vi "util.load.test.cases.vi"(11 "String":string) -> (3 "Array":T1[](array[typedef]))   [LabVIEW 2021]
uses:
  Test.Case.type.ctl
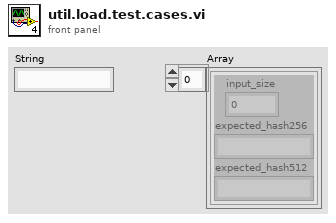
[diagram p1: front panel]
types:
  T1 = typedef "Test.Case.type.ctl" = cluster{"input_size":i32, "expected_hash256":string, "expected_hash512":string}
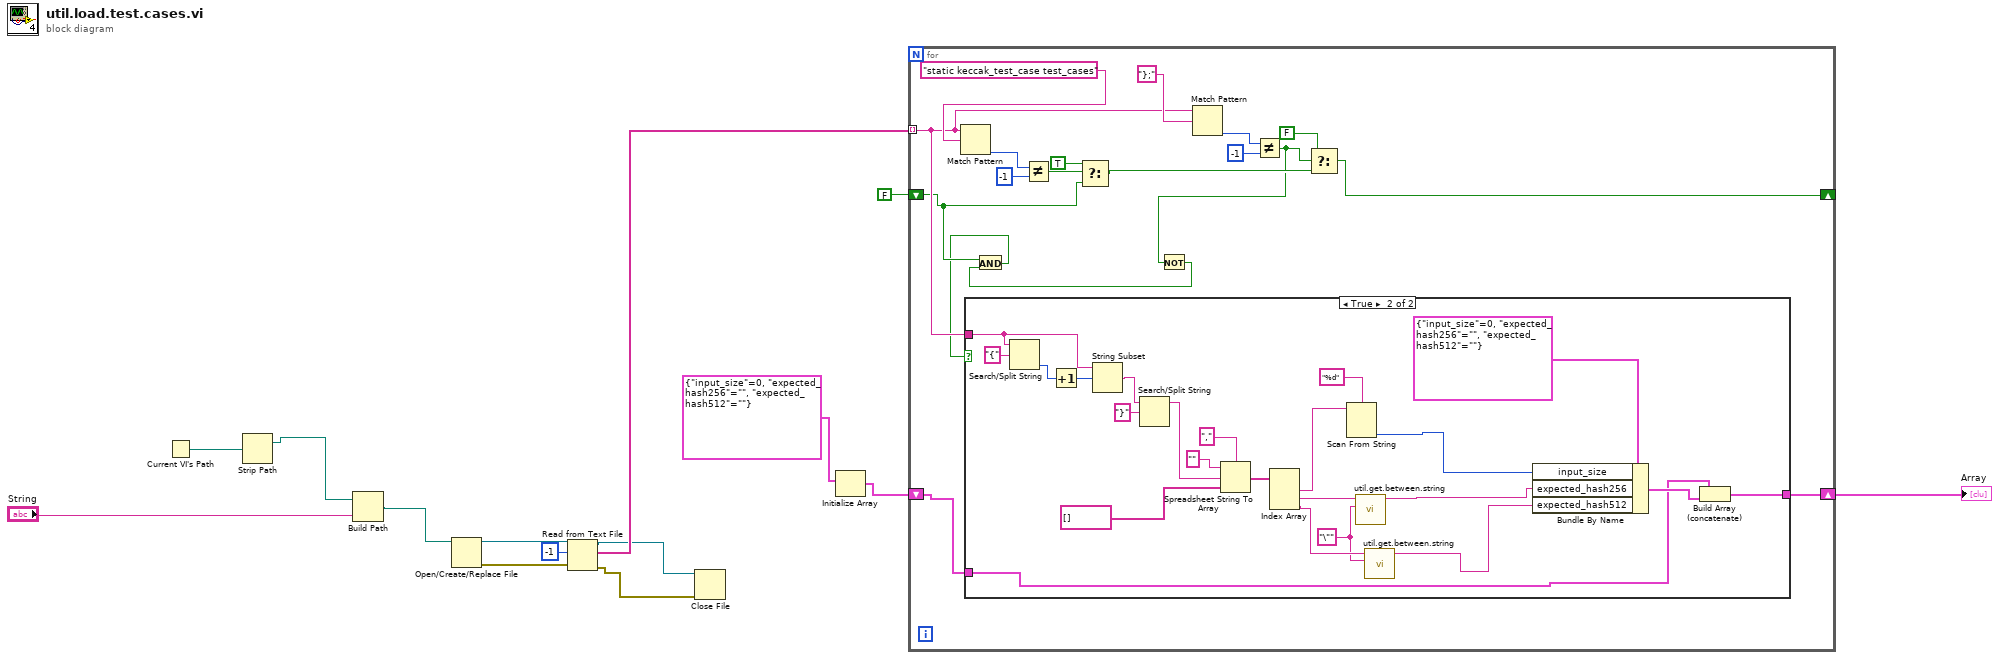
[diagram p0: block diagram]
diagram:
  n1 = Current VI's Path() -> (path=w7:path)
  n2 = Strip Path(path=w7) -> (stripped path=w8:path)  [unwired: 1 out]
  n3 = Build Path(base path=w8, name or relative path="String") -> (appended path=w2:path)
  n4 = Open/Create/Replace File(file path (use dialog)=w2) -> (refnum out=w3:refnum<file>, error out=w5:errorcluster)  [unwired: 5 in, 1 out]
  n5 = Read from Text File(file (use dialog)=w3, count=-1, error in=w5) -> (refnum out=w4:refnum<file>, text=w10:string[], error out=w6:errorcluster)  [unwired: 1 in, 1 out]
  n6 = Close File(refnum=w4, error in=w6) -> ()  [unwired: 2 out]
  n7 = Initialize Array(T1 {"input_size"=0, "expected_hash256"="", "expected_hash512"=""}) -> (w12:T1[])  [unwired: 1 in]
  n8 = for {
    tunnel: w10 -> [w26] mode=indexing
    shift-right: [w22] -> _
    shift-left: FALSE -> [w20]
    shift-right: [w16] -> w14
    shift-left: w12 -> [w15]
    n9 = Match Pattern(string=w26, regular expression="static keccak_test_case test_cases") -> (offset past match=w31:i32)  [unwired: 1 in, 3 out]
    n10 = Not Equal?(x=w31, y=-1) -> (x != y?=w29:bool)
    n11 = Select(t=TRUE, s=w29, f=w20) -> (s? t:f=w23:bool)
    n12 = Match Pattern(string=w26, regular expression="};") -> (offset past match=w25:i32)  [unwired: 1 in, 3 out]
    n13 = Not Equal?(x=w25, y=-1) -> (x != y?=w18:bool)
    n14 = Not(x=w18) -> (.not. x?=w17:bool)
    n15 = And(x=w20, y=w17) -> (x .and. y?=w19:bool)
    n16 = case shown="True" w19 {
      tunnel: w26 -> [_ w53]
      tunnel: [w33 w35] -> w16
      tunnel: w15 -> [w33 w34]
      frame False {
      }
      frame True {
        w41 = "\"" ("search string/char (-)")
        n17 = Search/Split String(string=w53, search string/char (-)="{") -> (offset of match=w55:i32)  [unwired: 1 in, 2 out]
        n18 = Increment(x=w55) -> (x+1=w54:i32)
        n19 = String Subset(string=w53, offset (0)=w54) -> (substring=w51:string)  [unwired: 1 in]
        n20 = Search/Split String(string=w51, search string/char (-)="}") -> (substring before match=w50:string)  [unwired: 1 in, 2 out]
        n21 = Spreadsheet String To Array(delimiter (Tab)=",", format string="", spreadsheet string=w50, array type (2D Dbl)=string[] []) -> (array=w46:string[])
        n22 = Index Array(array=w46) -> (element #1=w45:string, element #2=w43:string, element #3=w42:string)  [unwired: 3 in]
        n23 = Scan From String(format string="%d", input string=w45) -> (output 1=w37:i32)  [unwired: 3 in, 3 out]
        n24 = call "util.get.between.string.vi"("search string/char (-)"=w41, "String in"=w43) -> ("String out"=w38:string)  [unwired: 9 in]
        n25 = call "util.get.between.string.vi"("search string/char (-)"=w41, "String in"=w42) -> ("String out"=w39:string)  [unwired: 9 in]
        n26 = Bundle By Name(cluster=T1 {"input_size"=0, "expected_hash256"="", "expected_hash512"=""}, "input_size"=w37, "expected_hash256"=w38, "expected_hash512"=w39) -> (w36:T1)
        n27 = Build Array (concatenate)(w34, w36) -> (w35:T1[])
      }
    }
    n28 = Select(t=FALSE, s=w18, f=w23) -> (s? t:f=w22:bool)
  }
  "Array" <- w14
